vi "Day_File_Plotter.vi"() -> ()   [LabVIEW 2022 SP3]
uses:
  Anemometry/Anemometry Sub Vis/File/Setup_Filetype.ctl
  ADAM Server/ADAM_Global.vi
panel:
  out "Update Time scales":bool
  out "All Plot Names":string[](array[string])
  in  "History (Hours)":i32 min=0
  in  "Use Full Files":bool
  in  "Reload":bool
  out "Setup exists?":bool
  out "Plot 1 status":string
  out "Change Scale?":bool
  out "Min Memory":timestamp
  out "Max Memory":timestamp
  in  "Show Full Time?":bool
  in  "Max Time":timestamp format="%<%H:%M\n%x>T"
  in  "Min Time":timestamp format="%<%H:%M\n%x>T"
  out "Plot 3 Chs":string[](array[string])
  out "Plot 2 Chs":string[](array[string])
  out "Plot 1 Chs":string[](array[string])
  in  "Save plot number":T1(ring)
  in  "Data folder location":path
  in  "Save 3":bool
  in  "Save 2":bool
  in  "Save 1":bool
  in  "Averaging Time (min)":dbl=0.01 min=0.0 step=0.01 format="%#.2f"
  in  "End Time":timestamp format="%<%H:%M\n%x>T"
  in  "Selector 1":i32[](listbox)
  in  "Search 1":string
  in  "Search 2":string
  in  "Search 3":string
  out "Last Updated":string
  out "Plot 3":cluster{"Times":dbl[], "Output array":dbl[]}[](graph)
  in  "Selector 3":i32[](listbox)
  out "Plot 2":cluster{"Times":dbl[], "Output array":dbl[]}[](graph)
  in  "Selector 2":i32[](listbox)
  in  "stop":bool
  out "Plot 1":cluster{dbl[], "Output array":dbl[]}[](graph)
  in  "History (days)":i32 min=0
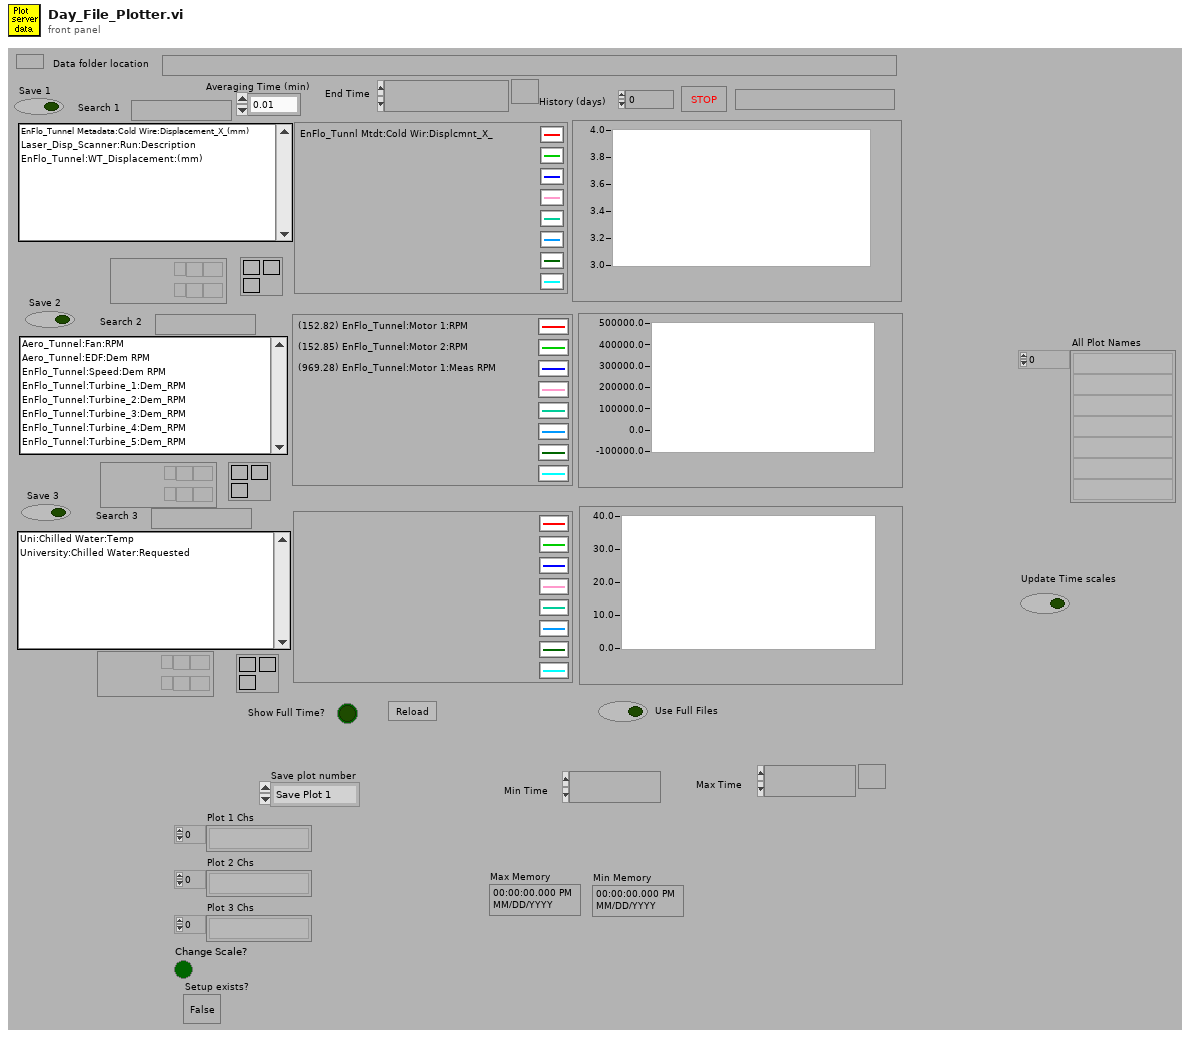
[diagram p1: front panel]
types:
  T1 = enum16{"Save Plot 1", "Save Plot 2", "Save Plot 3"}
  T2 = typedef "Setup_Filetype.ctl" = enum16{"Measurement Setups", "Calibration Setups", "General", "Results File Plotter Setups", "Speed Calib Tweaks"}
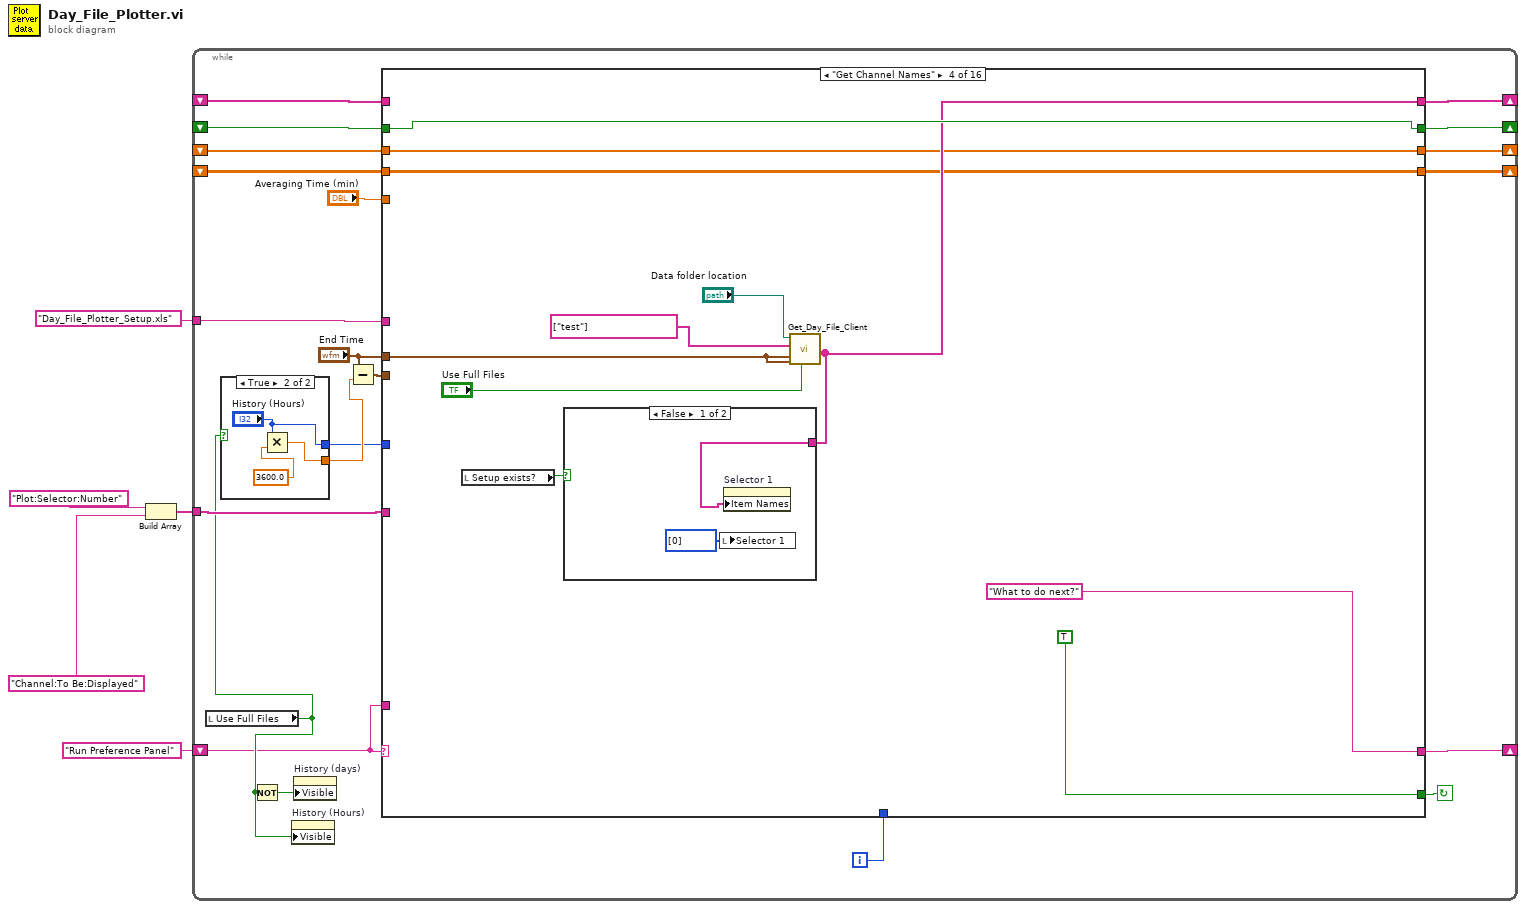
[diagram p0: block diagram]
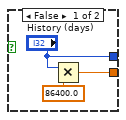
[diagram p2: hidden frame]
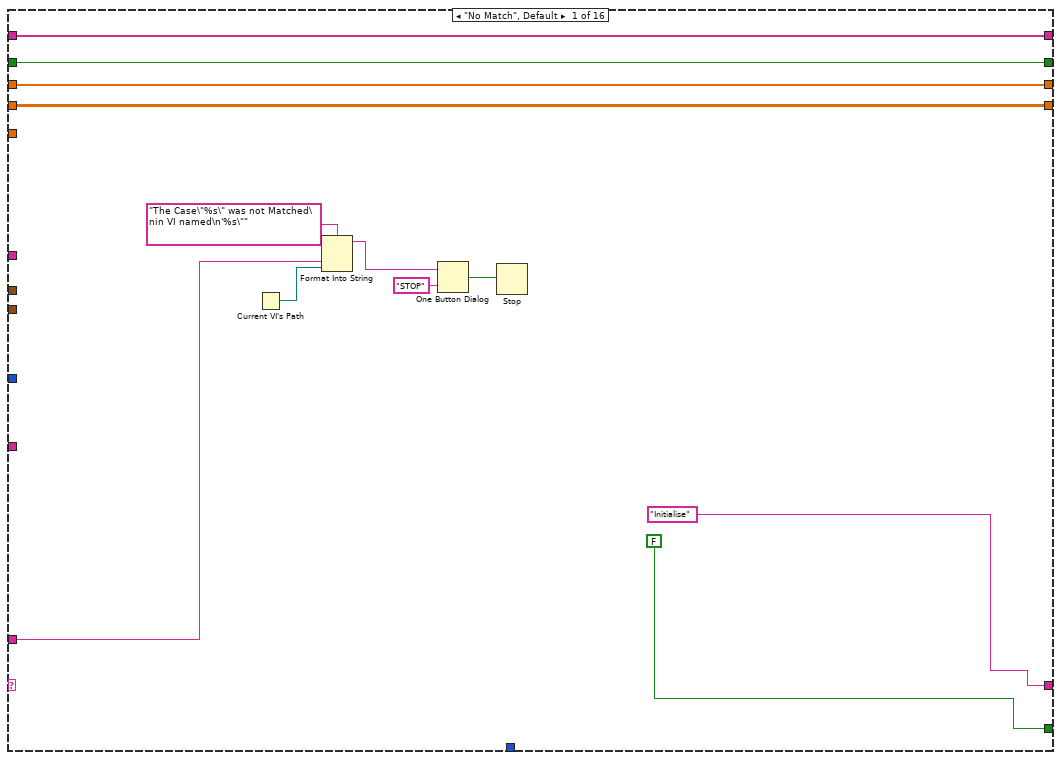
[diagram p3: hidden frame]
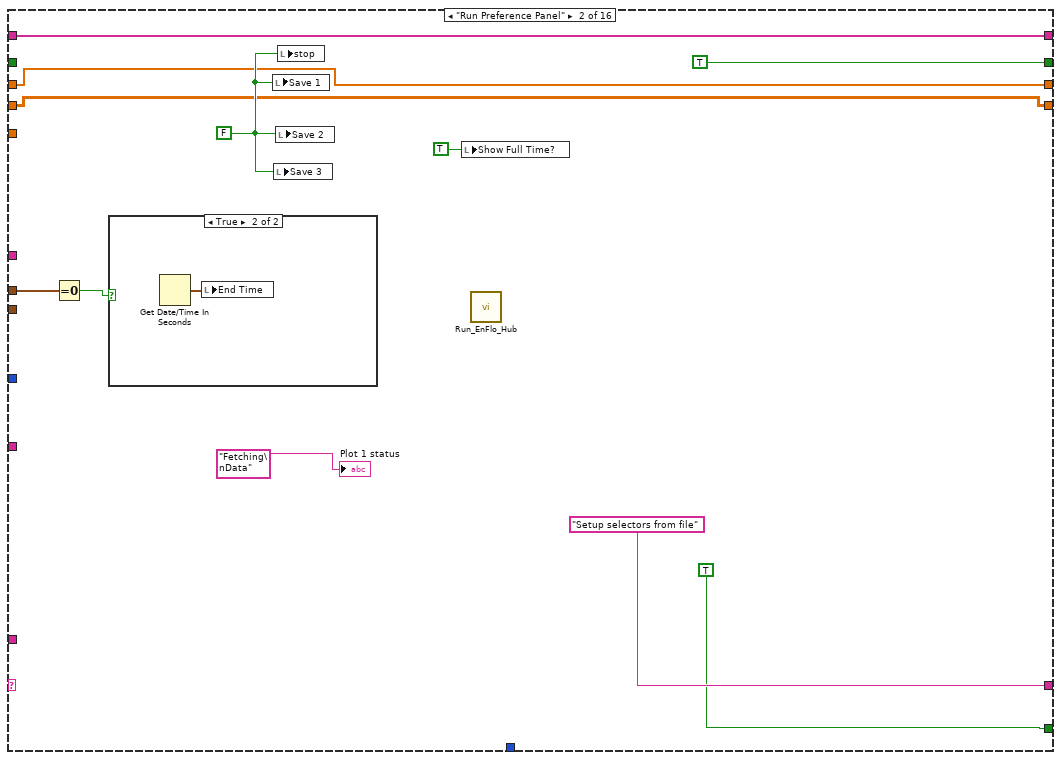
[diagram p4: hidden frame]
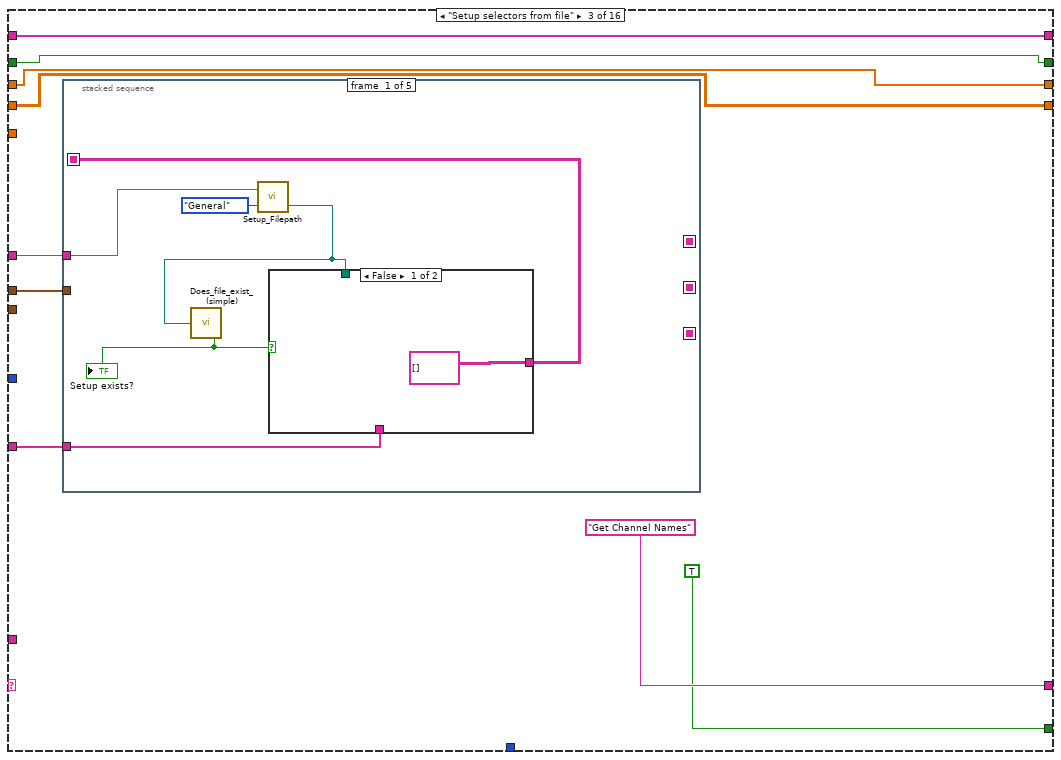
[diagram p6: hidden frame]
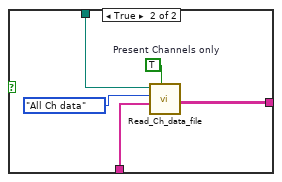
[diagram p7: hidden frame]
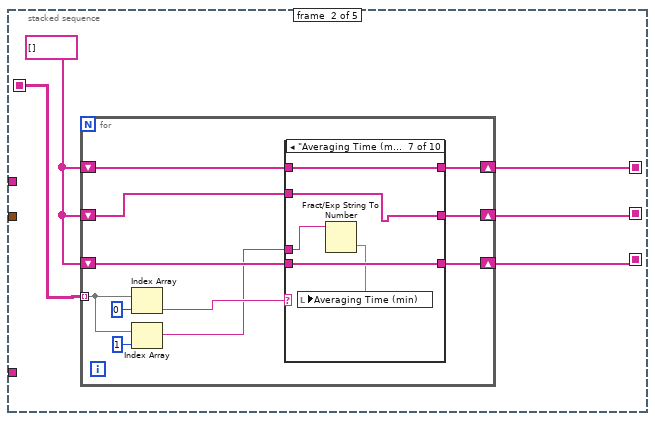
[diagram p8: hidden frame]
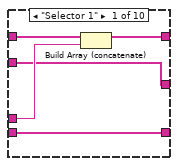
[diagram p9: hidden frame]
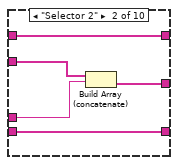
[diagram p10: hidden frame]
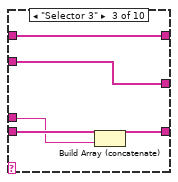
[diagram p11: hidden frame]
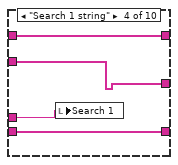
[diagram p12: hidden frame]
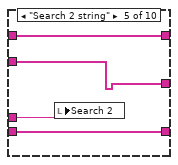
[diagram p13: hidden frame]
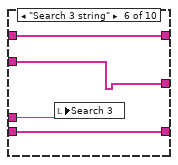
[diagram p14: hidden frame]
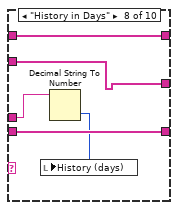
[diagram p15: hidden frame]
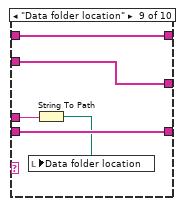
[diagram p16: hidden frame]
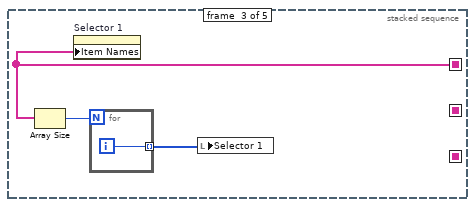
[diagram p18: hidden frame]
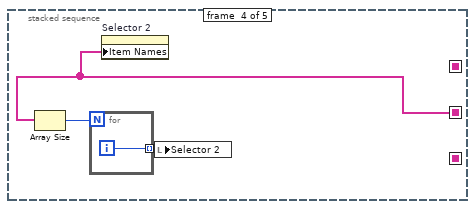
[diagram p19: hidden frame]
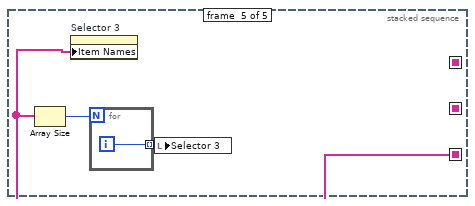
[diagram p20: hidden frame]
diagram:
  n1 = Build Array("Plot:Selector:Number", "Channel:To Be:Displayed") -> (w2:string[])
  n2 = while {
    shift-left: "Run Preference Panel" -> [w11]
    shift-right: [w25] -> _
    tunnel: w2 -> [w24]
    tunnel: "Day_File_Plotter_Setup.xls" -> [w23]
    shift-right: [w19] -> _
    shift-left: _ -> [w18]
    shift-right: [w15] -> _
    shift-left: _ -> [w14]
    shift-right: [w10] -> _
    shift-left: _ -> [w9]
    shift-right: [w8] -> _
    shift-left: _ -> [w7]
    i -> [w6]
    stop <- w26 continue-if-true
    n3 = local read "Use Full Files"() -> (w12:bool)
    n4 = case shown="True" w12 {
      tunnel: [w28 w31] -> w22
      tunnel: ["History (days)" "History (Hours)"] -> w17
      frame False {
        n5 = Multiply(x="History (days)", y=86400.0) -> (x*y=w28:dbl)
      }
      frame True {
        n6 = Multiply(x="History (Hours)", y=3600.0) -> (x*y=w31:dbl)
      }
    }
    n7 = Not(x=w12) -> (.not. x?=w13:bool)
    n8 = property on="History (Hours)" class="DigNum (strict)"("Visible"=w12) -> ()  [unwired: 2 in, 2 out]
    n9 = property on="History (days)" class="DigNum (strict)"("Visible"=w13) -> ()  [unwired: 2 in, 2 out]
    n10 = Subtract(x="End Time", y=w22) -> (x-y=w21:timestamp)
    n11 = case shown="\"Get Channel Names\"" w11 {
      tunnel: [FALSE TRUE TRUE TRUE TRUE TRUE TRUE TRUE TRUE TRUE TRUE TRUE TRUE TRUE TRUE w663] -> w26
      tunnel: ["Initialise" "Setup selectors from file" "Get Channel Names" "What to do next?" "Plot1" "Plot2" "Plot3" "Rescale plots?" "Update Plot1?" w346 w401 w457 w510 w614 w642 "Check for Zoom" ("t")] -> w25
      tunnel: w11 -> [w39 _ _ _ _ _ _ _ _ _ _ _ _ _ _ _]
      tunnel: w24 -> [_ _ w62 _ _ _ _ _ _ _ _ _ _ _ _ w669]
      tunnel: w23 -> [_ _ w63 _ _ _ _ _ _ _ _ _ _ _ _ w668]
      tunnel: w21 -> [_ _ _ _ w180 _ _ _ _ _ _ _ _ _ _ _]
      tunnel: "End Time" -> [_ w52 w60 w158 w179 _ _ _ _ _ _ _ _ w607 _ _]
      tunnel: [w36 TRUE w61 w159 w183 w207 w242 w277 w307 w359 w415 w470 w511 w606 w641 w666] -> w19
      tunnel: w18 -> [w36 _ w61 w159 w183 w207 w242 w277 w307 w359 w415 w470 w511 _ w640 w666]
      tunnel: w17 -> [_ _ _ _ _ _ _ _ _ _ _ _ _ w594 _ w661]
      tunnel: "Averaging Time (min)" -> [_ _ _ _ w182 _ _ _ _ _ _ _ _ w605 _ w665]
      tunnel: [w35 w50 w59 w155 w176 w193 w228 w268 w308 w355 w411 w466 w512 w603 w647 w664] -> w15
      tunnel: w14 -> [w35 w50 w59 _ w177 w193 w228 w268 w308 w355 w411 w466 w512 w603 w647 w664]
      tunnel: [w34 w46 w58 w152 w165 w198 w231 w267 w301 w343 w399 w454 w508 w593 w639 w659] -> w10
      tunnel: w9 -> [w34 w46 w58 w152 _ w198 w231 w267 w301 w343 w399 w454 w508 w593 w639 w659]
      tunnel: [w33 w45 w57 w151 w169 w195 w232 w263 w300 w342 w398 w453 w507 w592 w638 w658] -> w8
      tunnel: w7 -> [w33 w45 w57 w151 _ w195 w232 w263 w300 w342 w398 w453 w507 w592 w638 w658]
      tunnel: w6 -> [_ _ _ _ _ _ _ _ _ _ _ _ _ w588 _ _]
      frame "No Match", Default {
        n12 = Current VI's Path() -> (path=w38:path)
        n13 = Format Into String(format string="The Case\"%s\" was not Matched\nin VI named\n'%s\"" ("Format String"), w39, w38) -> (resulting string=w42:string)  [unwired: 2 in, 1 out]
        n14 = One Button Dialog(message=w42, button name ("OK")="STOP") -> (true=w40:bool)
        n15 = Stop(stop? (T)=w40) -> ()
      }
      frame "Run Preference Panel" {
        w49 = FALSE
        n16 = Equal To 0?(x=w52) -> (x = 0?=w51:bool)
        n17 = case shown="True" w51 {
          frame False {
          }
          frame True {
            n18 = Get Date/Time In Seconds() -> (seconds since 1Jan1904=w56:timestamp)
            n19 = local write "End Time"(w56) -> ()
          }
        }
        n20 = local write "Save 1"(w49) -> ()
        n21 = local write "Save 3"(w49) -> ()
        n22 = local write "Save 2"(w49) -> ()
        n23 = local write "stop"(w49) -> ()
        n24 = local write "Show Full Time?"(TRUE ("Show Full Time?")) -> ()
        n25 = call "Run_EnFlo_Hub.vi"() -> ()  [unwired: 1 in, 7 out]
        "Plot 1 status" <- "Fetching\nData" ("Plot 1 status")
      }
      frame "Setup selectors from file" {
        n26 = stacked-sequence {
          seq-local: [w70 _ _ _ _] -> [_ w82 _ _ _]
          seq-local: [_ w80 _ _ _] -> [_ _ w141 _ _]
          seq-local: [_ w78 _ _ _] -> [_ _ _ w143 _]
          seq-local: [_ w79 _ _ _] -> [_ _ _ _ w147]
          tunnel: w63 -> [w67 _ _ _ _]
          tunnel: w62 -> [w71 _ _ _ _]
          tunnel: w60 -> [_ _ _ _ _]
          frame #0 {
            n27 = call "Setup_Filepath.vi"("Setup File Type"=Setup_Filetype."General", "Filename in"=w67) -> ("Filename Out"=w66:path)  [unwired: 1 out]
            n28 = call "Does_file_exist_(simple).vi"("Pathname"=w66) -> ("exists?"=w69:bool)
            "Setup exists?" <- w69
            n29 = case shown="False" w69 {
              tunnel: w66 -> [_ w77]
              tunnel: w71 -> [_ w76]
              tunnel: [string[][] [] ("Channel Values") w73] -> w70
              frame False {
              }
              frame True {
                w75 = TRUE  # Present Channels only
                n30 = call "Read_Ch_data_file.vi"("Present Channels only"=w75, "Present Channels"=w76, "Output"=enum16{"All Ch data", "The last few rows"}."All Ch data", "Filename"=w77) -> ("Channel Values"=w73:string[][])  [unwired: 1 in, 4 out]
              }
            }
          }
          frame #1 {
            w81 = string[] []
            n31 = for {
              shift-right: [w88] -> w80
              shift-left: w81 -> [w89]
              tunnel: w82 -> [w90] mode=indexing
              shift-right: [w86] -> w78
              shift-left: w81 -> [w87]
              shift-right: [w84] -> w79
              shift-left: w81 -> [w85]
              n32 = Index Array(array=w90, index=0 ("Index")) -> (element=w92:string)
              n33 = Index Array(array=w90, index=1 ("Index")) -> (element=w83:string)
              n34 = case shown="\"Averaging Time (min)\"" w92 {
                tunnel: w89 -> [w98 w103 w104 w112 w116 w120 w125 w126 w133 w138]
                tunnel: [w97 w103 w104 w112 w116 w120 w125 w126 w133 w138] -> w88
                tunnel: w83 -> [w96 w100 w106 w109 w113 w117 w122 w128 w132 _]
                tunnel: w87 -> [w95 w101 w105 w111 w115 w119 w124 w130 w135 w137]
                tunnel: [w95 w99 w105 w111 w115 w119 w124 w130 w135 w137] -> w86
                tunnel: w85 -> [w94 w102 w108 w110 w114 w118 w123 w129 w134 w136]
                tunnel: [w94 w102 w107 w110 w114 w118 w123 w129 w134 w136] -> w84
                frame "Selector 1" {
                  n35 = Build Array (concatenate)(w98, w96) -> (w97:string[])
                }
                frame "Selector 2" {
                  n36 = Build Array (concatenate)(w101, w100) -> (w99:string[])
                }
                frame "Selector 3" {
                  n37 = Build Array (concatenate)(w108, w106) -> (w107:string[])
                }
                frame "Search 1 string" {
                  n38 = local write "Search 1"(w109) -> ()
                }
                frame "Search 2 string" {
                  n39 = local write "Search 2"(w113) -> ()
                }
                frame "Search 3 string" {
                  n40 = local write "Search 3"(w117) -> ()
                }
                frame "Averaging Time (min)" {
                  n41 = Fract/Exp String To Number(string=w122) -> (number=w121:dbl)  [unwired: 3 in, 1 out]
                  n42 = local write "Averaging Time (min)"(w121) -> ()
                }
                frame "History in Days" {
                  n43 = Decimal String To Number(string=w128) -> (number=w127:i32)  [unwired: 3 out]
                  n44 = local write "History (days)"(w127) -> ()
                }
                frame "Data folder location" {
                  n45 = String To Path(string=w132) -> (path=w131:path)
                  n46 = local write "Data folder location"(w131) -> ()
                }
                frame "No match", Default {
                }
              }
            }
          }
          frame #2 {
            n47 = Array Size(array=w141) -> (size(s)=w140:i32)
            n48 = property on="Selector 1" class="LstBox (strict)"("Item Names"=w141) -> ()  [unwired: 2 in, 2 out]
            n49 = for {
              N: w140 -> [_]
              tunnel: [w142] -> w139 mode=indexing
              i -> [w142]
            }
            n50 = local write "Selector 1"(w139) -> ()
          }
          frame #3 {
            n51 = Array Size(array=w143) -> (size(s)=w145:i32)
            n52 = for {
              N: w145 -> [_]
              tunnel: [w146] -> w144 mode=indexing
              i -> [w146]
            }
            n53 = property on="Selector 2" class="LstBox (strict)"("Item Names"=w143) -> ()  [unwired: 2 in, 2 out]
            n54 = local write "Selector 2"(w144) -> ()
          }
          frame #4 {
            n55 = Array Size(array=w147) -> (size(s)=w149:i32)
            n56 = property on="Selector 3" class="LstBox (strict)"("Item Names"=w147) -> ()  [unwired: 2 in, 2 out]
            n57 = for {
              N: w149 -> [_]
              tunnel: [w150] -> w148 mode=indexing
              i -> [w150]
            }
            n58 = local write "Selector 3"(w148) -> ()
          }
        }
      }
      frame "Get Channel Names" {
        n59 = local read "Setup exists?"() -> (w154:bool)
        n60 = call "Get_Day_File_Client.vi"("Use Full Res Files"="Use Full Files", "End time"=w158, "Start time"=w158, "Channel Names"=string[] ["test"], "Data folder location"="Data folder location") -> ("All Channel Names"=w155:string[])  [unwired: 2 in, 4 out]
        n61 = case shown="False" w154 {
          tunnel: w155 -> [w163 _]
          frame False {
            n62 = local write "Selector 1"(i32[] [0] ("Selector 1")) -> ()
            n63 = property on="Selector 1" class="LstBox (strict)"("Item Names"=w163) -> ()  [unwired: 2 in, 2 out]
          }
          frame True {
          }
        }
      }
      frame "Get Data from Files" {
        n64 = local read "Data folder location"() -> (w181:path)
        n65 = local read "Plot 2 Chs"() -> (w172:string[])
        n66 = local read "Plot 3 Chs"() -> (w171:string[])
        n67 = local read "Plot 1 Chs"() -> (w173:string[])
        n68 = property on="Plot 1 status" class="Str"("Visible"=TRUE) -> ()  [unwired: 2 in, 2 out]
        n69 = Build Array (concatenate)(w173, w172, w171) -> (w170:string[])
        n70 = call "Analyse_string_array.vi"("String array"=w170) -> ("Unique strings"=w167:string[])  [unwired: 1 in, 1 out]
        "All Plot Names" <- w167
        n71 = local read "Use Full Files"() -> (w174:bool)
        n72 = call "Get_Day_File_Client.vi"("Use Full Res Files"=w174, "Averaging Time (min)"=w182, "End time"=w179, "Start time"=w180, "Channel Names"=w167, "Data folder location"=w181) -> ("All Channel Names"=w168:string[], "Data"=w164:dbl[][], "Times"=w169:dbl[])  [unwired: 1 in, 2 out]
        n73 = Array Size(array=w168) -> (size(s)=w178:i32)
        n74 = Equal To 0?(x=w178) -> (x = 0?=w175:bool)
        n75 = Select(t=w177, s=w175, f=w168) -> (s? t:f=w176:string[])
        n76 = case shown="False" w175 {
          tunnel: w169 -> [w192 _]
          frame False {
            n77 = Array Max & Min(array=w192) -> (max value=w191:dbl, min value=w190:dbl)  [unwired: 2 out]
            n78 = To Time Stamp(1:w191) -> (0:→"Max Memory":timestamp)
            n79 = To Time Stamp(1:w190) -> (0:→"Min Memory":timestamp)
          }
          frame True {
          }
        }
        n80 = flat-sequence {
          tunnel: [w187] -> w165
          tunnel: w164 -> [w187]
          frame #0 {
            n81 = property on="Plot 1 status" class="Str"("Visible"=FALSE) -> ()  [unwired: 2 in, 2 out]
          }
        }
      }
      frame "Plot1" {
        n82 = local read "Plot 1 Chs"() -> (w196:string[])
        n83 = local read "All Plot Names"() -> (w197:string[])
        n84 = for {
          tunnel: w197 -> [w212]
          tunnel: w196 -> [w211] mode=indexing
          tunnel: [w210] -> w194 mode=indexing
          n85 = Search 1D Array(1D array=w212, element=w211) -> (index of element=w210:i32)  [unwired: 1 in]
        }
        n86 = for {
          tunnel: w198 -> [w215]
          tunnel: [w225] -> w206 mode=indexing
          tunnel: w195 -> [w224]
          tunnel: [w220] -> w199 mode=indexing
          tunnel: w196 -> [w217] mode=indexing
          tunnel: w194 -> [w214] mode=indexing
          n87 = Index Array(array=w215, index (row)=w214) -> (element=w213:dbl[])  [unwired: 1 in]
          n88 = Bundle("Times"=w224, "Data"=w213) -> (w225:cluster{"Times":dbl[], "Data":dbl[]})  [unwired: 1 out]
          n89 = call "Mean_fr_NaN_data for any fraction.vi"("Data"=w213) -> ("Mean value"=w216:dbl)
          n90 = call "Number_2_string.vi"("precision"="2", "number"=w216) -> ("String"=w218:string)
          n91 = Format Into String(format string="(%s) %s", w218, w217) -> (resulting string=w221:string)  [unwired: 2 in, 1 out]
          n92 = call "Abbreviate_string.vi"("Input String"=w221, "Max String Length"=40) -> ("Output String"=w220:string)  [unwired: 1 in, 2 out]
        }
        "Plot 1" <- w206
        n93 = Array Size(array=w199) -> (size(s)=w204:i32)
        n94 = Subtract(x=10 ("dimension size"), y=w204) -> (x-y=w205:i32)
        n95 = Initialize Array("", w205) -> (w202:string[])
        n96 = Build Array (concatenate)(w199, w202) -> (w200:string[])
        n97 = for {
          tunnel: w200 -> [w226] mode=indexing
          i -> [w227]
          n98 = property on="Plot 1" class="XYGraph (strict)"("Active Plot"=w227, "Plot.Plot Name"=w226) -> ()  [unwired: 2 in, 2 out]
        }
      }
      frame "Plot2" {
        n99 = local read "Plot 2 Chs"() -> (w229:string[])
        n100 = local read "All Plot Names"() -> (w233:string[])
        n101 = for {
          tunnel: w233 -> [w247]
          tunnel: w229 -> [w246] mode=indexing
          tunnel: [w245] -> w230 mode=indexing
          n102 = Search 1D Array(1D array=w247, element=w246) -> (index of element=w245:i32)  [unwired: 1 in]
        }
        n103 = for {
          tunnel: [w260] -> w235 mode=indexing
          tunnel: w232 -> [w259]
          tunnel: [w255] -> w234 mode=indexing
          tunnel: w229 -> [w252] mode=indexing
          tunnel: w231 -> [w250]
          tunnel: w230 -> [w249] mode=indexing
          n104 = Index Array(array=w250, index (row)=w249) -> (element=w248:dbl[])  [unwired: 1 in]
          n105 = Bundle("Times"=w259, "Data"=w248) -> (w260:cluster{"Times":dbl[], "Data":dbl[]})  [unwired: 1 out]
          n106 = call "Mean_fr_NaN_data for any fraction.vi"("Data"=w248) -> ("Mean value"=w251:dbl)
          n107 = call "Number_2_string.vi"("precision"="2", "number"=w251) -> ("String"=w253:string)
          n108 = Format Into String(format string="(%s) %s", w253, w252) -> (resulting string=w256:string)  [unwired: 2 in, 1 out]
          n109 = call "Abbreviate_string.vi"("Input String"=w256, "Max String Length"=40) -> ("Output String"=w255:string)  [unwired: 1 in, 2 out]
        }
        "Plot 2" <- w235
        n110 = Array Size(array=w234) -> (size(s)=w240:i32)
        n111 = Subtract(x=10 ("dimension size"), y=w240) -> (x-y=w241:i32)
        n112 = Initialize Array("", w241) -> (w238:string[])
        n113 = Build Array (concatenate)(w234, w238) -> (w236:string[])
        n114 = for {
          tunnel: w236 -> [w261] mode=indexing
          i -> [w262]
          n115 = property on="Plot 2" class="XYGraph (strict)"("Active Plot"=w262, "Plot.Plot Name"=w261) -> ()  [unwired: 2 in, 2 out]
        }
      }
      frame "Plot3" {
        n116 = local read "Plot 3 Chs"() -> (w265:string[])
        n117 = local read "All Plot Names"() -> (w266:string[])
        n118 = for {
          tunnel: w266 -> [w282]
          tunnel: w265 -> [w281] mode=indexing
          tunnel: [w280] -> w264 mode=indexing
          n119 = Search 1D Array(1D array=w282, element=w281) -> (index of element=w280:i32)  [unwired: 1 in]
        }
        n120 = for {
          tunnel: [w295] -> w270 mode=indexing
          tunnel: w263 -> [w294]
          tunnel: [w290] -> w269 mode=indexing
          tunnel: w265 -> [w287] mode=indexing
          tunnel: w267 -> [w285]
          tunnel: w264 -> [w284] mode=indexing
          n121 = Index Array(array=w285, index (row)=w284) -> (element=w283:dbl[])  [unwired: 1 in]
          n122 = Bundle("Times"=w294, "Data"=w283) -> (w295:cluster{"Times":dbl[], "Data":dbl[]})  [unwired: 1 out]
          n123 = call "Mean_fr_NaN_data for any fraction.vi"("Data"=w283) -> ("Mean value"=w286:dbl)
          n124 = call "Number_2_string.vi"("precision"="2", "number"=w286) -> ("String"=w288:string)
          n125 = Format Into String(format string="(%s) %s", w288, w287) -> (resulting string=w291:string)  [unwired: 2 in, 1 out]
          n126 = call "Abbreviate_string.vi"("Input String"=w291, "Max String Length"=40) -> ("Output String"=w290:string)  [unwired: 1 in, 2 out]
        }
        "Plot 3" <- w270
        n127 = Array Size(array=w269) -> (size(s)=w275:i32)
        n128 = Subtract(x=10 ("dimension size"), y=w275) -> (x-y=w276:i32)
        n129 = Initialize Array("", w276) -> (w273:string[])
        n130 = Build Array (concatenate)(w269, w273) -> (w271:string[])
        n131 = for {
          tunnel: w271 -> [w296] mode=indexing
          i -> [w297]
          n132 = property on="Plot 3" class="XYGraph (strict)"("Active Plot"=w297, "Plot.Plot Name"=w296) -> ()  [unwired: 2 in, 2 out]
        }
      }
      frame "Check for Zoom" {
        n133 = local read "Change Scale?"() -> (w303:bool)
        n134 = Or(x=w303, y="Show Full Time?") -> (x .or. y?=w302:bool)
        n135 = case shown="True" w302 {
          tunnel: [w309 TRUE] -> w298
          frame False {
            n136 = local read "Min Time"() -> (w319:timestamp)
            n137 = local read "Max Time"() -> (w318:timestamp)
            n138 = To Double Precision Float(number=w318) -> (double precision float=w314:dbl)
            n139 = To Double Precision Float(number=w319) -> (double precision float=w313:dbl)
            n140 = for {
              N: 3 -> [_]
              shift-right: [w327] -> w311
              shift-left: w314 -> [w326]
              shift-right: [w323] -> w312
              shift-left: w313 -> [w324]
              tunnel: [w320] -> w310 mode=indexing
              i -> [w330]
              n141 = Increment(x=w330) -> (x+1=w329:i32)
              n142 = case shown="3" w329 {
                tunnel: [w333 w335 w338] -> w328
                tunnel: [w332 w334 w337] -> w325
                tunnel: [TRUE TRUE FALSE] -> _
                frame 1, Default {
                  n143 = property on="Plot 1" class="XYGraph (strict)"() -> ("X Scale.Range:Maximum"=w333:dbl, "X Scale.Range:Minimum"=w332:dbl)  [unwired: 2 in, 2 out]
                }
                frame 2 {
                  n144 = property on="Plot 2" class="XYGraph (strict)"() -> ("X Scale.Range:Maximum"=w335:dbl, "X Scale.Range:Minimum"=w334:dbl)  [unwired: 2 in, 2 out]
                }
                frame 3 {
                  n145 = property on="Plot 3" class="XYGraph (strict)"() -> ("X Scale.Range:Maximum"=w338:dbl, "X Scale.Range:Minimum"=w337:dbl)  [unwired: 2 in, 2 out]
                }
              }
              n146 = Less?(x=w328, y=w326) -> (x < y?=w322:bool)
              n147 = Greater?(x=w325, y=w324) -> (0:w321:bool)
              n148 = Select(t=w328, s=w322, f=w326) -> (s? t:f=w327:dbl)
              n149 = Select(t=w325, s=w321, f=w324) -> (s? t:f=w323:dbl)
              n150 = Or(x=w322, y=w321) -> (x .or. y?=w320:bool)
            }
            n151 = To Time Stamp(1:w311) -> (0:w316:timestamp)
            n152 = To Time Stamp(1:w312) -> (0:w317:timestamp)
            n153 = Or Array Elements(Boolean array=w310) -> (logical OR=w309:bool)
            n154 = local write "Min Time"(w317) -> ()
            n155 = local write "Max Time"(w316) -> ()
          }
          frame True {
          }
        }
        "Update Time scales" <- w298
        n156 = Wait For Front Panel Activity(1:300 ("timeout ms (-1 never timeout)")) -> ()  [unwired: 2 in, 1 out]
      }
      frame "Update Plot1?" {
        n157 = property on="Selector 1" class="LstBox (strict)"() -> ("Item Names"=w353:string[])  [unwired: 2 in, 2 out]
        n158 = case shown="True" "Save 1" {
          tunnel: ["Update Plot2?" "Save Plot" ("t")] -> w344
          frame False {
          }
          frame True {
            n159 = local write "Save plot number"(T1."Save Plot 1" ("Save plot number")) -> ()
          }
        }
        n160 = for {
          tunnel: w355 -> [w386]
          shift-right: [w381] -> w354
          shift-left: string[] [] -> [w382]
          tunnel: w353 -> [w384]
          tunnel: "Selector 1" -> [w383] mode=indexing
          n161 = Index Array(array=w384, index=w383) -> (element=w380:string)
          n162 = Search 1D Array(1D array=w386, element=w380) -> (index of element=w385:i32)  [unwired: 1 out]
          n163 = case shown="0, Default" w385 {
            tunnel: w385 -> [_ _]
            tunnel: w382 -> [w389 w390]
            tunnel: [w388 w390] -> w381
            tunnel: w380 -> [w387 _]
            frame 0, Default {
              n164 = Build Array (concatenate)(w389, w387) -> (w388:string[])
            }
            frame -1 {
            }
          }
        }
        "Plot 1 Chs" <- w354
        n165 = while {
          shift-right: [w391] -> w362
          shift-left: _ -> [w396]
          tunnel: [w396] -> w361
          shift-right: [w393] -> _
          shift-left: _ -> [w394]
          tunnel: w359 -> [w393]
          tunnel: [w392] -> w358
          tunnel: w354 -> [w391]
          stop <- FALSE continue-if-true
          n166 = Not Equal?(x=w394, y=w393) -> (x != y?=w392:bool)
        }
        n167 = Not Equal?(x=w361, y=w362) -> (x != y?=w360:bool)
        n168 = And(x=w359, y=w358) -> (x .and. y?=w357:bool)
        n169 = Compound Arithmetic op=OR(w357, w360) -> (w345:bool)
        n170 = case shown="True" w345 {
          tunnel: [w368 "Get Data from Files"] -> w346
          tunnel: w344 -> [w368 _]
          frame False {
          }
          frame True {
            n171 = property on="Plot 1 status" class="Str"("Visible"=TRUE) -> ()  [unwired: 2 in, 2 out]
          }
        }
        n172 = call "Selection_with_Search.vi"("Selected Channel Names"=w354, "Search String"="Search 1", "All Channel Names"=w355) -> ("Item Names"=w350:string[])
        n173 = for {
          tunnel: w350 -> [w379]
          tunnel: w354 -> [w378] mode=indexing
          tunnel: [w377] -> w351 mode=indexing
          n174 = Search 1D Array(1D array=w379, element=w378) -> (index of element=w377:i32)  [unwired: 1 out]
        }
        n175 = local read "Update Time scales"() -> (w341:bool)
        n176 = Not Equal?(x=w350, y=w353) -> (x != y?=w352:bool)
        n177 = case shown="True" w352 {
          tunnel: w351 -> [_ w376]
          tunnel: w350 -> [_ w375]
          frame False {
          }
          frame True {
            n178 = local write "Selector 1"(w376) -> ()
            n179 = property on="Selector 1" class="LstBox (strict)"("Item Names"=w375, "Top Row"=0) -> ()  [unwired: 2 in, 2 out]
          }
        }
        n180 = case shown="True" w341 {
          frame False {
          }
          frame True {
            n181 = To Double Precision Float(number="Max Time") -> (double precision float=w366:dbl)
            n182 = To Double Precision Float(number="Min Time") -> (double precision float=w364:dbl)
            n183 = property on="Plot 1" class="XYGraph (strict)"("X Scale.Range:Maximum"=w366, "X Scale.Range:Minimum"=w364) -> ()  [unwired: 2 in, 2 out]
          }
        }
      }
      frame "Update Plot2?" {
        n184 = property on="Selector 2" class="LstBox (strict)"() -> ("Item Names"=w406:string[])  [unwired: 2 in, 2 out]
        n185 = case shown="True" "Save 2" {
          tunnel: ["Update Plot3?" "Save Plot" ("t")] -> w400
          frame False {
          }
          frame True {
            n186 = local write "Save plot number"(T1."Save Plot 2" ("Save plot number")) -> ()
          }
        }
        n187 = for {
          tunnel: w411 -> [w441]
          shift-right: [w436] -> w410
          shift-left: string[] [] -> [w437]
          tunnel: w406 -> [w439]
          tunnel: "Selector 2" -> [w438] mode=indexing
          n188 = Index Array(array=w439, index=w438) -> (element=w435:string)
          n189 = Search 1D Array(1D array=w441, element=w435) -> (index of element=w440:i32)  [unwired: 1 out]
          n190 = case shown="0, Default" w440 {
            tunnel: w440 -> [_ _]
            tunnel: w437 -> [w444 w445]
            tunnel: [w443 w445] -> w436
            tunnel: w435 -> [w442 _]
            frame 0, Default {
              n191 = Build Array (concatenate)(w444, w442) -> (w443:string[])
            }
            frame -1 {
            }
          }
        }
        "Plot 2 Chs" <- w410
        n192 = while {
          shift-right: [w446] -> w418
          shift-left: _ -> [w451]
          tunnel: [w451] -> w417
          shift-right: [w448] -> _
          shift-left: _ -> [w449]
          tunnel: w415 -> [w448]
          tunnel: [w447] -> w414
          tunnel: w410 -> [w446]
          stop <- FALSE continue-if-true
          n193 = Not Equal?(x=w449, y=w448) -> (x != y?=w447:bool)
        }
        n194 = Not Equal?(x=w417, y=w418) -> (x != y?=w416:bool)
        n195 = And(x=w415, y=w414) -> (x .and. y?=w413:bool)
        n196 = Compound Arithmetic op=OR(w413, w416) -> (w402:bool)
        n197 = case shown="True" w402 {
          tunnel: [w424 "Get Data from Files"] -> w401
          tunnel: w400 -> [w424 _]
          frame False {
          }
          frame True {
            (unwired) TRUE ("Visible")
          }
        }
        n198 = call "Selection_with_Search.vi"("Selected Channel Names"=w410, "Search String"="Search 2", "All Channel Names"=w411) -> ("Item Names"=w407:string[])
        n199 = for {
          tunnel: w407 -> [w434]
          tunnel: w410 -> [w433] mode=indexing
          tunnel: [w432] -> w408 mode=indexing
          n200 = Search 1D Array(1D array=w434, element=w433) -> (index of element=w432:i32)  [unwired: 1 out]
        }
        n201 = local read "Update Time scales"() -> (w397:bool)
        n202 = Not Equal?(x=w407, y=w406) -> (x != y?=w409:bool)
        n203 = case shown="True" w409 {
          tunnel: w408 -> [_ w431]
          tunnel: w407 -> [_ w430]
          frame False {
          }
          frame True {
            n204 = local write "Selector 2"(w431) -> ()
            n205 = property on="Selector 2" class="LstBox (strict)"("Item Names"=w430, "Top Row"=0) -> ()  [unwired: 2 in, 2 out]
          }
        }
        n206 = case shown="True" w397 {
          frame False {
          }
          frame True {
            n207 = local read "Max Time"() -> (w422:timestamp)
            n208 = local read "Min Time"() -> (w423:timestamp)
            n209 = To Double Precision Float(number=w422) -> (double precision float=w421:dbl)
            n210 = To Double Precision Float(number=w423) -> (double precision float=w420:dbl)
            n211 = property on="Plot 2" class="XYGraph (strict)"("X Scale.Range:Maximum"=w421, "X Scale.Range:Minimum"=w420) -> ()  [unwired: 2 in, 2 out]
          }
        }
      }
      frame "Update Plot3?" {
        n212 = property on="Selector 3" class="LstBox (strict)"() -> ("Item Names"=w458:string[])  [unwired: 2 in, 2 out]
        n213 = case shown="True" "Save 3" {
          tunnel: ["Rescale plots?" "Save Plot" ("t")] -> w455
          frame False {
          }
          frame True {
            n214 = local write "Save plot number"(T1."Save Plot 3" ("Save plot number")) -> ()
          }
        }
        n215 = for {
          tunnel: w466 -> [w496]
          shift-right: [w491] -> w465
          shift-left: string[] [] -> [w492]
          tunnel: w458 -> [w494]
          tunnel: "Selector 3" -> [w493] mode=indexing
          n216 = Index Array(array=w494, index=w493) -> (element=w490:string)
          n217 = Search 1D Array(1D array=w496, element=w490) -> (index of element=w495:i32)  [unwired: 1 out]
          n218 = case shown="0, Default" w495 {
            tunnel: w495 -> [_ _]
            tunnel: w492 -> [w499 w500]
            tunnel: [w498 w500] -> w491
            tunnel: w490 -> [w497 _]
            frame 0, Default {
              n219 = Build Array (concatenate)(w499, w497) -> (w498:string[])
            }
            frame -1 {
            }
          }
        }
        "Plot 3 Chs" <- w465
        n220 = while {
          shift-right: [w501] -> w473
          shift-left: _ -> [w506]
          tunnel: [w506] -> w472
          shift-right: [w503] -> _
          shift-left: _ -> [w504]
          tunnel: w470 -> [w503]
          tunnel: [w502] -> w469
          tunnel: w465 -> [w501]
          stop <- FALSE continue-if-true
          n221 = Not Equal?(x=w504, y=w503) -> (x != y?=w502:bool)
        }
        n222 = Not Equal?(x=w472, y=w473) -> (x != y?=w471:bool)
        n223 = And(x=w470, y=w469) -> (x .and. y?=w468:bool)
        n224 = Compound Arithmetic op=OR(w468, w471) -> (w456:bool)
        n225 = case shown="True" w456 {
          tunnel: [w479 "Get Data from Files"] -> w457
          tunnel: w455 -> [w479 _]
          frame False {
          }
          frame True {
            (unwired) TRUE ("Visible")
          }
        }
        n226 = call "Selection_with_Search.vi"("Selected Channel Names"=w465, "Search String"="Search 3", "All Channel Names"=w466) -> ("Item Names"=w462:string[])
        n227 = for {
          tunnel: w462 -> [w489]
          tunnel: w465 -> [w488] mode=indexing
          tunnel: [w487] -> w463 mode=indexing
          n228 = Search 1D Array(1D array=w489, element=w488) -> (index of element=w487:i32)  [unwired: 1 out]
        }
        n229 = Not Equal?(x=w462, y=w458) -> (x != y?=w464:bool)
        n230 = local read "Update Time scales"() -> (w452:bool)
        n231 = case shown="True" w464 {
          tunnel: w463 -> [_ w486]
          tunnel: w462 -> [_ w485]
          frame False {
          }
          frame True {
            n232 = local write "Selector 3"(w486) -> ()
            n233 = property on="Selector 3" class="LstBox (strict)"("Item Names"=w485, "Top Row"=0) -> ()  [unwired: 2 in, 2 out]
          }
        }
        n234 = case shown="True" w452 {
          frame False {
          }
          frame True {
            n235 = local read "Max Time"() -> (w477:timestamp)
            n236 = local read "Min Time"() -> (w478:timestamp)
            n237 = To Double Precision Float(number=w477) -> (double precision float=w476:dbl)
            n238 = To Double Precision Float(number=w478) -> (double precision float=w475:dbl)
            n239 = property on="Plot 3" class="XYGraph (strict)"("X Scale.Range:Maximum"=w476, "X Scale.Range:Minimum"=w475) -> ()  [unwired: 2 in, 2 out]
          }
        }
      }
      frame "Save Plot" {
        n240 = stacked-sequence {
          seq-local: [_ w534 _] -> [_ _ w569]
          seq-local: [_ w522 _] -> [_ _ w571]
          seq-local: [_ w520 _] -> [_ _ w570]
          seq-local: [w513 _ _] -> [_ _ w561]
          tunnel: [_ "What to do next?" _] -> w510
          frame #0 {
            n241 = File Dialog(7:"Please provide a file name" ("prompt")) -> (3:w519:path)  [unwired: 1 in, 8 out]
            n242 = Strip Path(path=w519) -> (stripped path=w517:path, name=w518:string)
            n243 = call "Add_filename_suffix.vi"("Filename"=w518, "Suffix to add"=".xls") -> ("Filename out"=w516:string)  [unwired: 3 out]
            n244 = Build Path(base path=w517, name or relative path=w516) -> (appended path=w513:path)
          }
          frame #1 {
            n245 = case shown="\"Save Plot 2\"" "Save plot number" {
              tunnel: [w547 w550 w553] -> w539
              tunnel: [w546 w549 w552] -> w534
              frame "Save Plot 1" {
                n246 = local read "Plot 1 Chs"() -> (w546:string[])
                n247 = local write "Save 1"(FALSE ("Save 1")) -> ()
                n248 = local read "Plot 1"() -> (w547:cluster{dbl[], "Output array":dbl[]}[])
              }
              frame "Save Plot 2" {
                n249 = local read "Plot 2 Chs"() -> (w549:string[])
                n250 = local write "Save 2"(FALSE ("Save 1")) -> ()
                n251 = local read "Plot 2"() -> (w550:cluster{"Times":dbl[], "Output array":dbl[]}[])
              }
              frame "Save Plot 3" {
                n252 = local read "Plot 3 Chs"() -> (w552:string[])
                n253 = local write "Save 3"(FALSE ("Save 1")) -> ()
                n254 = local read "Plot 3"() -> (w553:cluster{"Times":dbl[], "Output array":dbl[]}[])
              }
            }
            n255 = local read "Min Time"() -> (w533:timestamp)
            n256 = local read "Max Time"() -> (w531:timestamp)
            n257 = Index Array(array=w539, index=0) -> (element=w537:cluster{"Times":dbl[], "Output array":dbl[]})
            n258 = To Double Precision Float(number=w533) -> (double precision float=w529:dbl)
            n259 = To Double Precision Float(number=w531) -> (double precision float=w530:dbl)
            n260 = Unbundle(w537) -> ("Times"=w523:dbl[])  [unwired: 1 out]
            n261 = Threshold 1D Array(2:w529, 3:w523) -> (0:w532:dbl)  [unwired: 1 out]
            n262 = Threshold 1D Array(2:w530, 3:w523) -> (0:w528:dbl)  [unwired: 1 out]
            n263 = Round Toward -Infinity(1:w532) -> (0:w526:dbl)
            n264 = Round Toward +Infinity(x=w528) -> (ceil(x): smallest int >= x=w527:dbl)
            n265 = To Long Integer(number=w526) -> (32bit integer=w525:i32)
            n266 = Subtract(x=w527, y=w526) -> (x-y=w524:dbl)
            n267 = for {
              N: w524 -> [_]
              tunnel: w525 -> [w544]
              tunnel: w523 -> [w542]
              tunnel: [w541] -> w522 mode=indexing
              tunnel: [w540] -> w521 mode=indexing
              i -> [w543]
              n268 = Add(x=w544, y=w543) -> (x+y=w540:i32)
              n269 = Index Array(array=w542, index=w540) -> (element=w541:dbl)
            }
            n270 = for {
              tunnel: w539 -> [w557] mode=indexing
              tunnel: w521 -> [w556]
              tunnel: [w554] -> w520 mode=indexing
              n271 = Unbundle(w557) -> ("Output array"=w555:dbl[])  [unwired: 1 out]
              n272 = for {
                tunnel: w556 -> [w560] mode=indexing
                tunnel: w555 -> [w559]
                tunnel: [w558] -> w554 mode=indexing
                n273 = Index Array(array=w559, index=w560) -> (element=w558:dbl)
              }
            }
          }
          frame #2 {
            w564 = FALSE  # append to file? (new file:F)
            n274 = for {
              tunnel: w570 -> [w583]
              tunnel: w571 -> [w577] mode=indexing
              tunnel: [w579] -> w563 mode=indexing
              i -> [w582]
              n275 = Number To Decimal String(number=w577) -> (decimal integer string=w578:string)  [unwired: 1 out]
              n276 = Index Array(array=w583, index (col)=w582) -> (element=w581:dbl[])  [unwired: 1 in]
              n277 = Get Date/Time String(seconds (now)=w577) -> (date string=w576:string, time string=w575:string)  [unwired: 2 out]
              n278 = for {
                tunnel: w581 -> [w585] mode=indexing
                tunnel: [w584] -> w580 mode=indexing
                n279 = call "Number_2_string.vi"("number"=w585) -> ("String"=w584:string)  [unwired: 1 in]
              }
              n280 = Build Array (concatenate)(w576, w575, w578, w580) -> (w579:string[])
            }
            n281 = Build Array (concatenate)("Date::", "Centre:Time:", "Seconds:Since:1st Jan 1904", w569) -> (w562:string[])
            n282 = call "Ch_names_to_rows.vi"("Channel Names"=w562) -> ("3 Row names"=w568:string[][])
            n283 = Build Array (concatenate)(w568, w563) -> (w566:string[][])
            n284 = Array To Spreadsheet String(array=w566, 3:"%s" ("format string")) -> (spreadsheet string=w565:string)  [unwired: 1 out]
            n285 = call "Write_File_Simple.vi"("append to file? (new file:F)"=w564, "character string"=w565, "file path"=w561) -> ()  [unwired: 2 out]
          }
        }
      }
      frame "What to do next?" {
        n286 = Get Date/Time String(date format (0)=enum16{"short", "long", "abbreviated"}."abbreviated") -> (date string=w610:string, time string=w611:string)  [unwired: 2 out]
        n287 = Concatenate Strings(w610, " at " ("Substring"), w611) -> (→"Last Updated":string)
        n288 = Array Size(array=w603) -> (size(s)=w604:i32)
        n289 = Greater Than 0?(x=w604) -> (x > 0?=w602:bool)
        n290 = Select(t="Check for Zoom", s=w602, f="Get Channel Names") -> (s? t:f=w599:string)
        n291 = Less?(x=w588, y=20) -> (x < y?=w586:bool)
        n292 = while {
          shift-right: [w617] -> _
          shift-left: _ -> [w634]
          shift-right: [w631] -> _
          shift-left: _ -> [w632]
          tunnel: w605 -> [w631]
          shift-right: [w629] -> _
          shift-left: _ -> [w630]
          tunnel: w607 -> [w629]
          tunnel: [w627] -> w606
          shift-right: [w625] -> w597
          shift-left: _ -> [w626]
          shift-right: [w619] -> _
          shift-left: _ -> [w620]
          tunnel: w594 -> [w617]
          tunnel: w586 -> [w616]
          stop <- FALSE continue-if-true
          n293 = local read "Use Full Files"() -> (w619:bool)
          n294 = Not Equal?(x=w617, y=w634) -> (x != y?=w624:bool)
          n295 = Not Equal?(x=w631, y=w632) -> (x != y?=w628:bool)
          n296 = Not Equal?(x=w630, y=w629) -> (x != y?=w623:bool)
          n297 = Not Equal?(x=w619, y=w620) -> (x != y?=w618:bool)
          n298 = Compound Arithmetic op=OR(w618, w624, w628, w623, "Reload") -> (w627:bool)
          n299 = case shown="False" w627 {
            tunnel: w626 -> [w635 w637]
            tunnel: [w636 w637] -> w625
            frame False {
              n300 = Increment(x=w635) -> (x+1=w636:dbl)
            }
            frame True {
            }
          }
          n301 = Compound Arithmetic op=OR(w624, w623, "Reload", w616) -> (→"Change Scale?":bool)
        }
        n302 = global read "ADAM_Global.vi" "stopAll"() -> (w589:bool)
        n303 = Quotient & Remainder(x=w597, y=500) -> (x-y*floor(x/y)=w596:i32)  [unwired: 1 out]
        n304 = Equal To 0?(x=w596) -> (x = 0?=w591:bool)
        n305 = Compound Arithmetic op=OR(w591, "stop", w589) -> (w595:bool)
        n306 = Select(t="Save Channel Names", s=w595, f=w599) -> (s? t:f=w614:string)
      }
      frame "Rescale plots?" {
        n307 = local read "Change Scale?"() -> (w645:bool)
        n308 = local read "Show Full Time?"() -> (w643:bool)
        n309 = Or(x=w645, y=w643) -> (x .or. y?=w644:bool)
        n310 = case shown="True" w644 {
          tunnel: ["What to do next?" "Update Plot1?"] -> w642
          tunnel: [w648 FALSE] -> w641
          tunnel: w640 -> [w648 _]
          frame False {
          }
          frame True {
            w651 = FALSE ("Show Full Time?")
            n311 = local write "Change Scale?"(w651) -> ()
            n312 = local write "Show Full Time?"(w651) -> ()
            n313 = local read "Max Memory"() -> (w653:timestamp)
            n314 = local read "Min Memory"() -> (w654:timestamp)
            n315 = local write "Max Time"(w653) -> ()
            n316 = local write "Min Time"(w654) -> ()
          }
        }
      }
      frame "Save Channel Names" {
        w660 = 10 ("y")
        n317 = Less?(x=w661, y=w660) -> (x < y?=w662:bool)
        n318 = stacked-sequence {
          seq-local: [w671 _ _] -> [_ w714 _]
          seq-local: [_ w711 _] -> [_ _ w725]
          tunnel: w669 -> [_ _ w726]
          tunnel: w668 -> [_ _ w722]
          tunnel: w665 -> [_ w710 _]
          tunnel: w662 -> [_ w698 _]
          tunnel: w661 -> [_ w697 _]
          tunnel: w660 -> [_ w696 _]
          frame #0 {
            n319 = for {
              N: 3 -> [_]
              shift-right: [w675] -> w671
              shift-left: string[][] [] -> [w677]
              i -> [w682]
              n320 = Increment(x=w682) -> (x+1=w679:i32)
              n321 = case shown="2" w679 {
                tunnel: [w689 w690 w692] -> w681
                tunnel: [w688 w691 w693] -> w673
                frame 1, Default {
                  n322 = local read "Selector 1"() -> (w689:i32[])
                  n323 = property on="Selector 1" class="LstBox (strict)"() -> ("Item Names"=w688:string[])  [unwired: 2 in, 2 out]
                }
                frame 2 {
                  n324 = local read "Selector 2"() -> (w690:i32[])
                  n325 = property on="Selector 2" class="LstBox (strict)"() -> ("Item Names"=w691:string[])  [unwired: 2 in, 2 out]
                }
                frame 3 {
                  n326 = local read "Selector 3"() -> (w692:i32[])
                  n327 = property on="Selector 3" class="LstBox (strict)"() -> ("Item Names"=w693:string[])  [unwired: 2 in, 2 out]
                }
              }
              n328 = Format Into String(format string="%d" ("Format String"), initial string="Selector ", w679) -> (resulting string=w676:string)  [unwired: 1 in, 1 out]
              n329 = for {
                tunnel: w681 -> [w687] mode=indexing
                tunnel: w676 -> [w686]
                tunnel: [w684] -> w674 mode=indexing
                tunnel: w673 -> [w683]
                n330 = Index Array(array=w683, index=w687) -> (element=w685:string)
                n331 = Build Array(w686, w685) -> (w684:string[])
              }
              n332 = Build Array (concatenate)(w677, w674) -> (w675:string[][])
            }
          }
          frame #1 {
            n333 = Select(t=w697, s=w698, f=w696) -> (s? t:f=w695:i32)
            n334 = local read "Data folder location"() -> (w701:path)
            n335 = local read "Search 1"() -> (w720:string)
            n336 = Number To Fractional String(number=w710, precision (6)=i16 2) -> (F-format string=w708:string)  [unwired: 2 in]
            n337 = local read "Search 2"() -> (w717:string)
            n338 = Number To Decimal String(number=w695) -> (decimal integer string=w705:string)  [unwired: 1 out]
            n339 = local read "Search 3"() -> (w716:string)
            n340 = Path To String(path=w701) -> (string=w700:string)
            n341 = Build Array("Averaging Time (min)" ("element"), w708) -> (w706:string[])
            n342 = Build Array("Search 1 string" ("element"), w720) -> (w707:string[])
            n343 = Build Array("History in Days" ("element"), w705) -> (w703:string[])
            n344 = Build Array("Search 2 string" ("element"), w717) -> (w713:string[])
            n345 = Build Array("Search 3 string" ("element"), w716) -> (w712:string[])
            n346 = Build Array("Data folder location", w700) -> (w699:string[])
            n347 = Build Array (concatenate)(w714, w699, w703, w706, w707, w713, w712) -> (w711:string[][])
          }
          frame #2 {
            n348 = call "Setup_Filepath.vi"("Setup File Type"=Setup_Filetype."General", "Filename in"=w722) -> ("Filename Out"=w721:path)  [unwired: 1 out]
            n349 = Array Size(array=w725) -> (size(s)=w728:i32[])
            n350 = Index Array(array=w728, index=1 ("Index")) -> (element=w727:i32)
            n351 = Not Equal To 0?(x=w727) -> (x != 0?=w724:bool)
            n352 = case shown="True" w724 {
              tunnel: w721 -> [w730 w735]
              tunnel: w725 -> [_ w736]
              tunnel: w726 -> [_ w737]
              frame False {
                n353 = Delete(path (use dialog)=w730) -> ()  [unwired: 1 in, 6 out]
              }
              frame True {
                w731 = FALSE  # append to file? (new file:F)
                n354 = call "Ch_names_to_rows.vi"("Channel Names"=w737) -> ("3 Row names"=w738:string[][])
                n355 = Build Array (concatenate)(w738, w736) -> (w733:string[][])
                n356 = Array To Spreadsheet String(array=w733, 3:"%s" ("format string")) -> (spreadsheet string=w732:string)  [unwired: 1 out]
                n357 = call "Write_File_Simple.vi"("append to file? (new file:F)"=w731, "character string"=w732, "file path"=w735) -> ()  [unwired: 2 out]
              }
            }
          }
        }
        n358 = global read "ADAM_Global.vi" "stopAll"() -> (w656:bool)
        n359 = local read "stop"() -> (w657:bool)
        n360 = Or(x=w656, y=w657) -> (x .or. y?=w655:bool)
        n361 = Not(x=w655) -> (.not. x?=w663:bool)
      }
    }
  }
